vi "tcpip_alone.vi"() -> ()   [LabVIEW 2020]
panel:
  in  "Boolean":bool
  in  "stop":bool
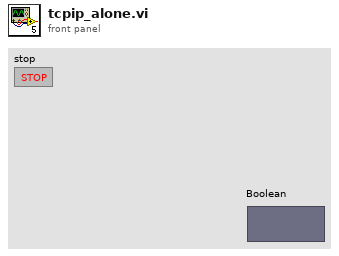
[diagram p1: front panel]
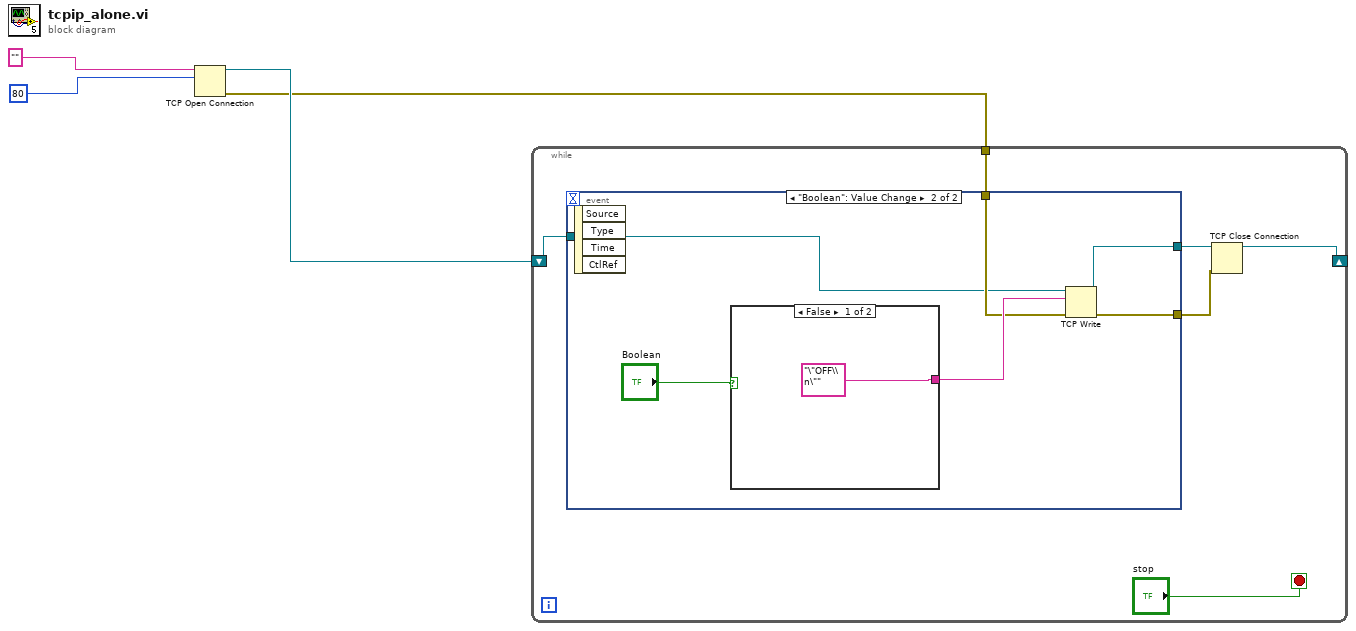
[diagram p0: block diagram]
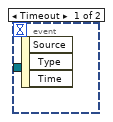
[diagram p2: hidden frame]
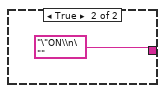
[diagram p3: hidden frame]
diagram:
  n1 = TCP Open Connection(address="", remote port or service name=u16 80) -> (connection ID=w2:refnum<k5>, error out=w1:errorcluster)  [unwired: 3 in]
  n2 = while {
    shift-right: [w5] -> _
    shift-left: w2 -> [w6]
    tunnel: w1 -> [w9]
    stop <- "stop" stop-if-true
    n3 = event shown="[1] \"Boolean\": Value Change" {
      selector: _ -> [_ _]
      dyn-events: _ -> [_ _]
      timeout: _ -> [_ _]
      tunnel: w9 -> [_ w15]
      tunnel: [_ w14] -> w8
      tunnel: [_ w13] -> w7
      tunnel: w6 -> [_ w12]
      event Timeout {
        n4 = event-data() -> ()  [unwired: 1 in, 3 out]
      }
      event "Boolean": Value Change {
        n5 = event-data() -> ()  [unwired: 1 in, 4 out]
        n6 = case shown="False" "Boolean" {
          tunnel: ["\"OFF\\n\"" "\"ON\\n\""] -> w16
          frame False {
          }
          frame True {
          }
        }
        n7 = TCP Write(connection ID=w12, data in=w16, error in (no error)=w15) -> (connection ID out=w13:refnum<k5>, error out=w14:errorcluster)  [unwired: 1 in, 1 out]
      }
    }
    n8 = TCP Close Connection(connection ID=w7, error in (no error)=w8) -> (connection ID out=w5:refnum<k5>)  [unwired: 1 in, 1 out]
  }
